vi "Close Target Config.vi"(8 "error in (no error)":errorcluster, 11 "Console Ref In":refnum<vi>) -> (0 "error out":errorcluster, 3 "Console Ref Out":refnum<vi>)   [LabVIEW 2015]
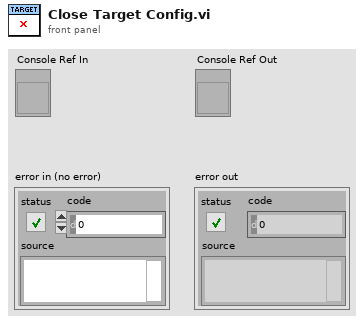
[diagram p1: front panel]
types:
  T1 = enum16{"open", "replace", "create", "open or create", "replace or create", "replace or create with confirmation"}
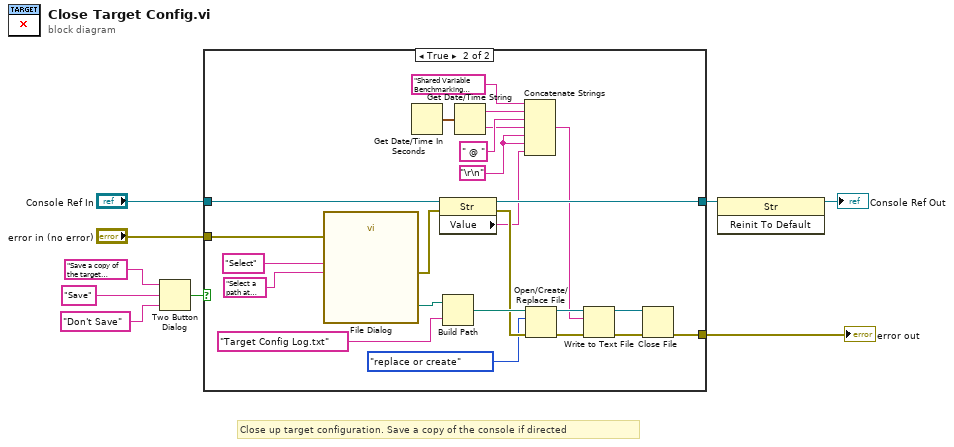
[diagram p0: block diagram]
diagram:
  # "Close up target configuration. Save a copy of the console if directed"
  n1 = Two Button Dialog(message="Save a copy of the target configuration console output?", 1:"Don't Save" ("F button name (\"Cancel\")"), 2:"Save") -> (T button?=w6:bool)
  n2 = case shown="True" w6 {
    tunnel: "error in (no error)" -> [w10 w35]
    tunnel: "Console Ref In" -> [w11 w32]
    tunnel: [w11 w24] -> w3
    tunnel: [w10 w13] -> w1
    frame False {
    }
    frame True {
      w21 = "\r\n"
      n3 = call "File Dialog"("prompt"="Select a path at which to save the configuration log file", "button label"="Select", "error in"=w35) -> ("selected path"=w30:path, "error out"=w31:errorcluster)  [unwired: 9 in, 2 out]
      n4 = Get Date/Time In Seconds() -> (seconds since 1Jan1904=w17:timestamp)
      n5 = property class="Str"(reference=w32, error in=w31) -> (reference out=w24:refnum<vi>, error out=w27:errorcluster, "Value"=w15:string)
      n6 = Build Path(base path=w30, name or relative path="Target Config Log.txt") -> (appended path=w28:path)
      n7 = Get Date/Time String(seconds (now)=w17) -> (date string=w18:string, time string=w19:string)  [unwired: 2 in]
      n8 = Concatenate Strings("Shared Variable Benchmarking Utility\n\nTarget Configuration Log -  ", w18, " @ ", w19, w21, w21, w15) -> (w14:string)
      n9 = Open/Create/Replace File(file path (use dialog)=w28, error in=w27, operation (0:open)=T1."replace or create") -> (refnum out=w26:refnum<file>, error out=w25:errorcluster)  [unwired: 3 in, 1 out]
      n10 = Write to Text File(file (use dialog)=w26, text=w14, error in=w25) -> (refnum out=w23:refnum<file>, error out=w22:errorcluster)  [unwired: 1 in, 1 out]
      n11 = Close File(refnum=w23, error in=w22) -> (error out=w13:errorcluster)  [unwired: 1 out]
    }
  }
  "error out" <- w1
  n12 = invoke class="Str" method="Reinit To Default"(reference=w3) -> (reference out=→"Console Ref Out":refnum<vi>)  [unwired: 2 in, 2 out]
